vi "Create reply queue (SubVI).vi"(3 "error in (no error)":errorcluster, 5 "Channel in":refnum<class "Channel.lvclass">) -> (0 "error out":errorcluster, 1 "Queue.lvclass":refnum<class "Queue.lvclass">, 2 "Channel out":refnum<class "Channel.lvclass">)   [LabVIEW 2016]
uses:
  <vilib>/Distrio/LabbitMQ/Channel/Channel.lvclass
  <vilib>/Distrio/LabbitMQ/Queue/Queue.lvclass
  <vilib>/Distrio/LabbitMQ/Channel/queue_declare_cluster.ctl
  global/Config_Infos.vi
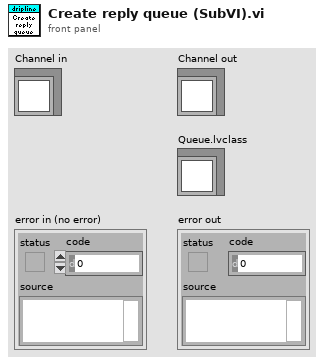
[diagram p1: front panel]
types:
  T1 = typedef "Channel.lvclass/queue_declare_cluster.ctl" = cluster{"queue":string, "durable (F)":bool, "exclusive (F)":bool, "autoDelete (F)":bool, "561934e089]], mscorlib, Version=0.0.0.0, Culture=neutral, PublicKeyToken=b77a5c561934e089\targuments":refnum<k24>}
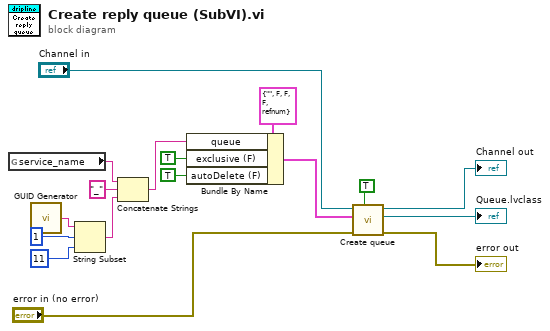
[diagram p0: block diagram]
diagram:
  n1 = global read "Config_Infos.vi" "service_name"() -> (w4:string)
  n2 = call "GUID Generator.vi"() -> ("GUID"=w6:string)  [unwired: 9 in]
  n3 = String Subset(string=w6, offset (0)=1, length (rest)=11 ("length (rest)")) -> (substring=w9:string)
  n4 = Concatenate Strings(w4, "_" ("string"), w9) -> (w10:string)
  n5 = Bundle By Name(cluster=T1 {"queue"="", "durable (F)"=FALSE, "exclusive (F)"=FALSE, "autoDelete (F)"=FALSE, "561934e089]], mscorlib, Version=0.0.0.0, Culture=neutral, PublicKeyToken=b77a5c561934e089\targuments"=refnum} ("QueueDeclare Properties"), "queue"=w10, "exclusive (F)"=TRUE, "autoDelete (F)"=TRUE) -> (w3:T1)
  n6 = call <vilib>:"Create queue.vi"("use QueueDeclareProperties (F)?"=TRUE, "error in (no error)"="error in (no error)", "QueueDeclare Properties"=w3, "Channel in"="Channel in") -> ("error out"=→"error out":errorcluster, "Queue.lvclass"=→"Queue.lvclass":refnum<class "Queue.lvclass">, "Channel out"=→"Channel out":refnum<class "Channel.lvclass">)  [unwired: 5 in]
